vi "20TVTI-Set-NV-Value.vi"(8 "error in (no error)":errorcluster, 10 "VTI Control":T1, 11 "Mercury Reference In":T2) -> (0 "error out":errorcluster)   [LabVIEW 2019]
uses:
  Equipment/Mercury iXX/Public/Controls/Mercury Reference.ctl
  Equipment/Mercury iXX/Public/Controls/Comms Transport Layer.ctl
  Equipment/Mercury iXX/Private/Controls/Query Dynamic Reference.ctl
  S16/VTI-control.ctl
  Equipment/Mercury iXX/Public/Libraries/Temperature/Open/Open Temperature Device.vi
  Equipment/Mercury iXX/Mercury iXX.lvlib
  Equipment/Mercury iXX/Public/Libraries/Temperature.lvlib
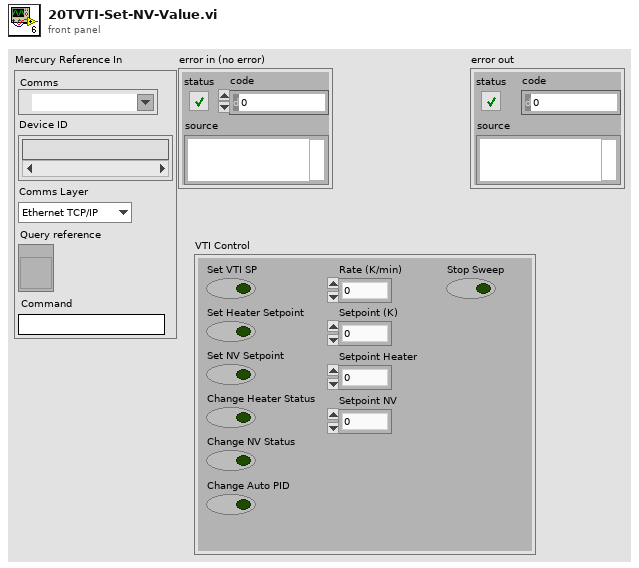
[diagram p1: front panel]
types:
  T1 = typedef "VTI-control.ctl" = cluster{"Set VTI SP":bool, "Change NV Status":bool, "Set NV Setpoint":bool, "Change Heater Status":bool, "Set Heater Setpoint":bool, "Setpoint (K)":dbl, "Rate (K/min)":dbl, "Setpoint Heater":dbl, "Setpoint NV":dbl, "Change Auto PID":bool, "Stop Sweep":bool}
  T2 = typedef "Mercury iXX.lvlib/Mercury Reference.ctl" = cluster{"Comms":refnum<visa-resource-name>, "Device ID":string[], "Comms Layer":T3, "Command":string, "Query reference":T4}
  T3 = typedef "Mercury iXX.lvlib/Comms Transport Layer.ctl" = enum16{"Ethernet TCP/IP", "USB", "ISOBus - RS-232", "GPIB"}
  T4 = typedef "Mercury iXX.lvlib/Query Dynamic Reference.ctl" = refnum<vi>
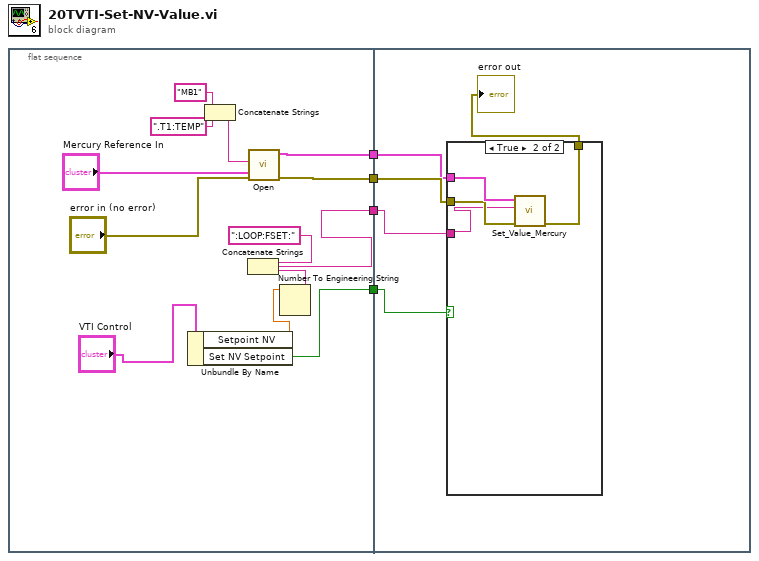
[diagram p0: block diagram]
diagram:
  n1 = flat-sequence {
    tunnel: [w17] -> w4
    tunnel: [w16] -> w3
    tunnel: [w9] -> w2
    tunnel: [w8] -> w1
    tunnel: w4 -> [w18]
    tunnel: w3 -> [w19]
    tunnel: w2 -> [w20]
    tunnel: w1 -> [w21]
    frame #0 {
      n2 = Unbundle By Name("VTI Control") -> ("Setpoint NV"=w14:dbl, "Set NV Setpoint"=w8:bool)
      n3 = Concatenate Strings("MB1", ".T1:TEMP" ("Device Identifier")) -> (w10:string)
      n4 = call-poly "Open.vi"("error in (no error)"="error in (no error)", "Device Identifier"=w10, "Mercury Reference In"="Mercury Reference In") -> ("error out"=w16:errorcluster, "Mercury Reference Out"=w17:T2)  [unwired: 2 in, 5 out]
      n5 = Number To Engineering String(4:w14) -> (0:w15:string)  [unwired: 3 in]
      n6 = Concatenate Strings(":LOOP:FSET:", w15) -> (w9:string)
    }
    frame #1 {
      n7 = case shown="True" w21 {
        tunnel: w18 -> [_ w27]
        tunnel: w19 -> [w23 w26]
        tunnel: [w23 w25] -> w22
        tunnel: w20 -> [_ w24]
        frame False {
        }
        frame True {
          n8 = call "Set_Value_Mercury.vi"("error in"=w26, "Noun(s)"=w24, "Mercury Reference In"=w27) -> ("error out"=w25:errorcluster)  [unwired: 7 in, 1 out]
        }
      }
      "error out" <- w22
    }
  }
